vi "Save_Single_Timetrace.vi"(1 "Headers":T1, 2 "Put each block into separate file":bool, 3 "Precision":i16=2, 7 "Index":i32, 9 "File Extension":string=".xls", 12 "Leave space between blocks?":bool, 14 "Separation Character":enum16{"Tab", "Comma"}(ring)) -> (4 "Plug in titles":string[](array[string]), 8 "Plug in values":string[](array[string]))   [LabVIEW 2021]
uses:
  Controls/Inst_type.ctl
  File/File Update Cluster.ctl
  Globals/Meas_global.vi
  Controls/File Header mode.ctl
panel:
  out "Output:Data File:Location":string
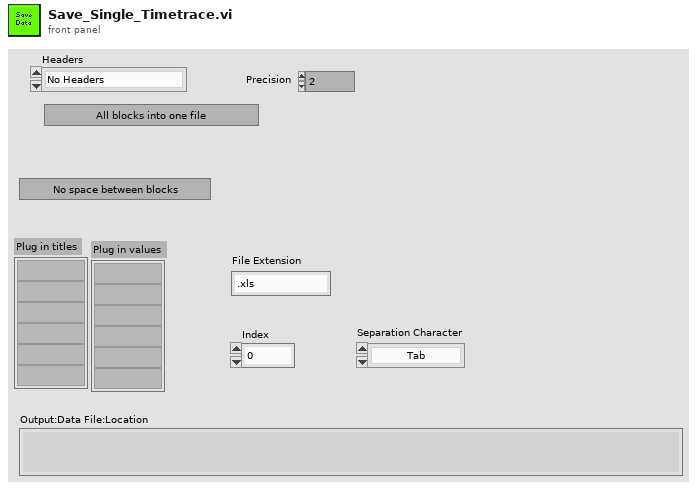
[diagram p1: front panel]
types:
  T1 = typedef "File Header mode.ctl" = enum16{"No Headers", "Headers in All files", "Separate Header File"}
  T2 = typedef "Analysis_info_cluster.ctl" = cluster{"Colour":u32, "Inst type":T3, "Inst name":string, "Symbol":string, "Code name":string, "Extra Info":string, "Inst Array":T4, "Extra Titles":string[], "Extra Values":string[], "U":dbl, "u^2":dbl, "u^3":dbl, "u^4":dbl, "Skew_u":dbl, "Kurt_u":dbl, "Sd Error in Mean":dbl, "% u'/U":dbl, "X":dbl, "Y":dbl, "Z":dbl, "Timescale integral Estimate":dbl, "Sd Error in Variance":dbl, "Calib File":path, "Calib Constants":dbl[], "Output Position":bool, "Stats":enum16{"None", "Basic", "Full"}, "Av Sampling Rate":dbl, "Av No of Samples":dbl, "Total Meas Time (s)":dbl, "ADAM Ch Name":string, "Max value":dbl, "Min value":dbl, "Req Sample Rate Hz":dbl, "Sync Delay Time (s)":dbl, "Ch No":i16, "Device":string, "Use Latest Calib":bool, "Port":string, "Metadata Ch Names":string[], "Metadata Ch Values":string[], "Label":string}
  T3 = typedef "Inst_type.ctl" = enum16{"Raw voltage", "Raw with zero offsetting", "Propeller anemometer", "Pressure Transducer", "Pitot-static tube", "Hot wire", "Cross wire 1", "Cross wire 2", "Generic Linear", "Generic Polynomial", "Generic BackPoly", "Fast FID", "Thermocouple", "Cold wire", "Pulsed Wire", "LDA Vel", "LDA Tran time", "LDA Arr time", "Microphone"}
  T4 = typedef "Instrument_Array.ctl" = enum16{"PWA", "LDA", "Analogue"}
  T5 = typedef "File Update Cluster.ctl" = cluster{"File Path":path, "Rows to Add":i32[], "Extra Ch Names":string[], "Extra Ch Values":string[], "Initial Header String":string, "Separation Character":enum16{"Tab", "Comma"}}
  T6 = typedef "Time_Trace_Cluster.ctl" = cluster{"Weighting":dbl[], "Voltage":dbl[], "Eng Values":dbl[]}
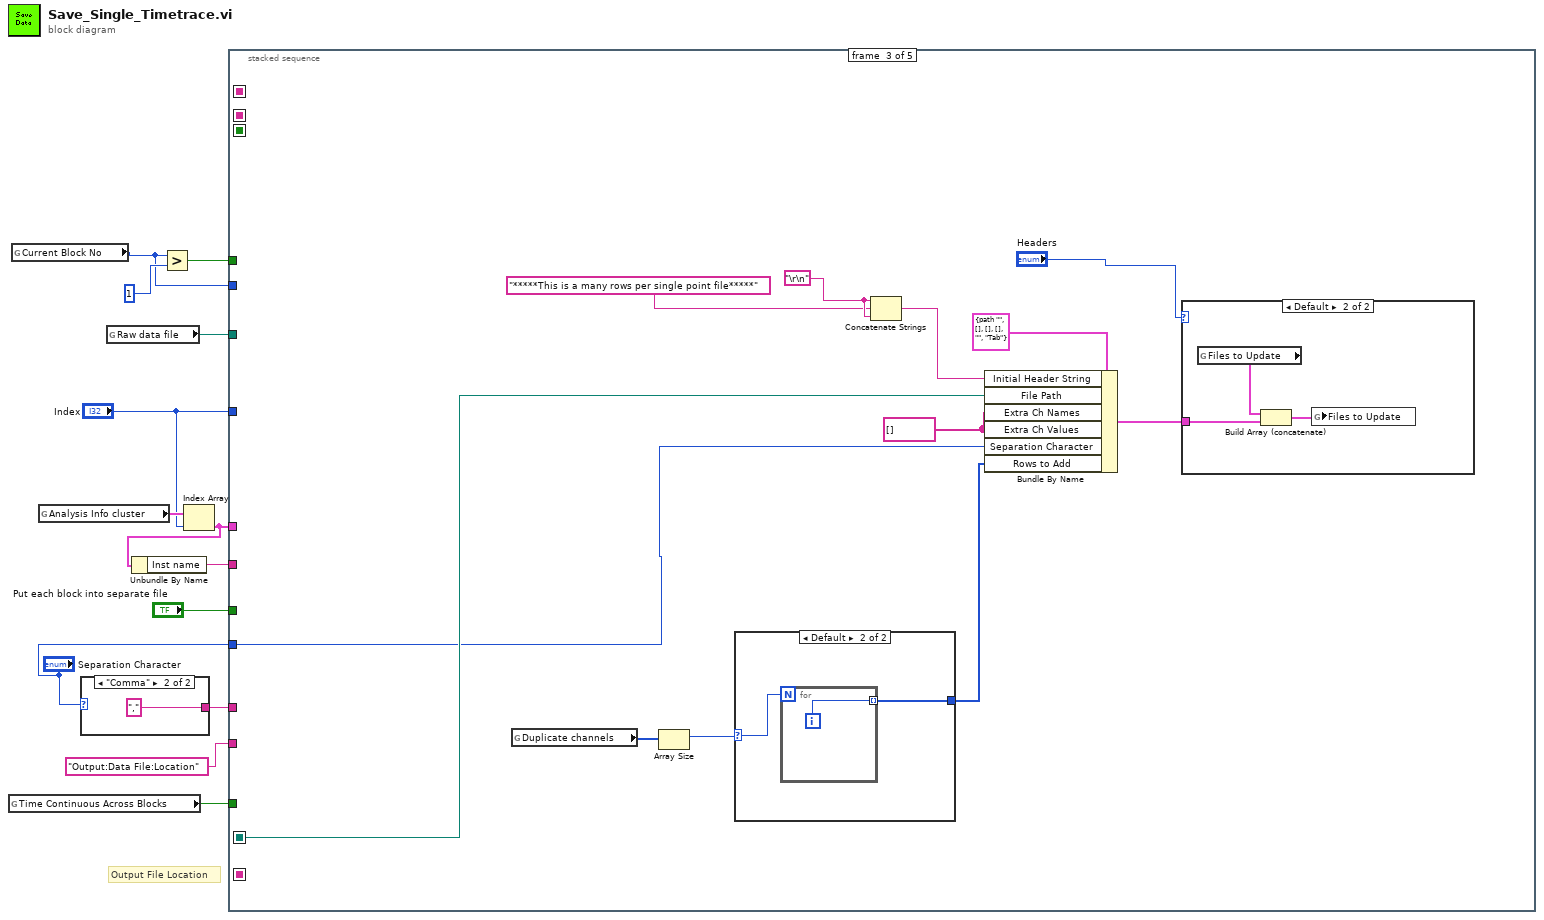
[diagram p0: block diagram]
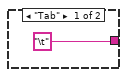
[diagram p2: hidden frame]
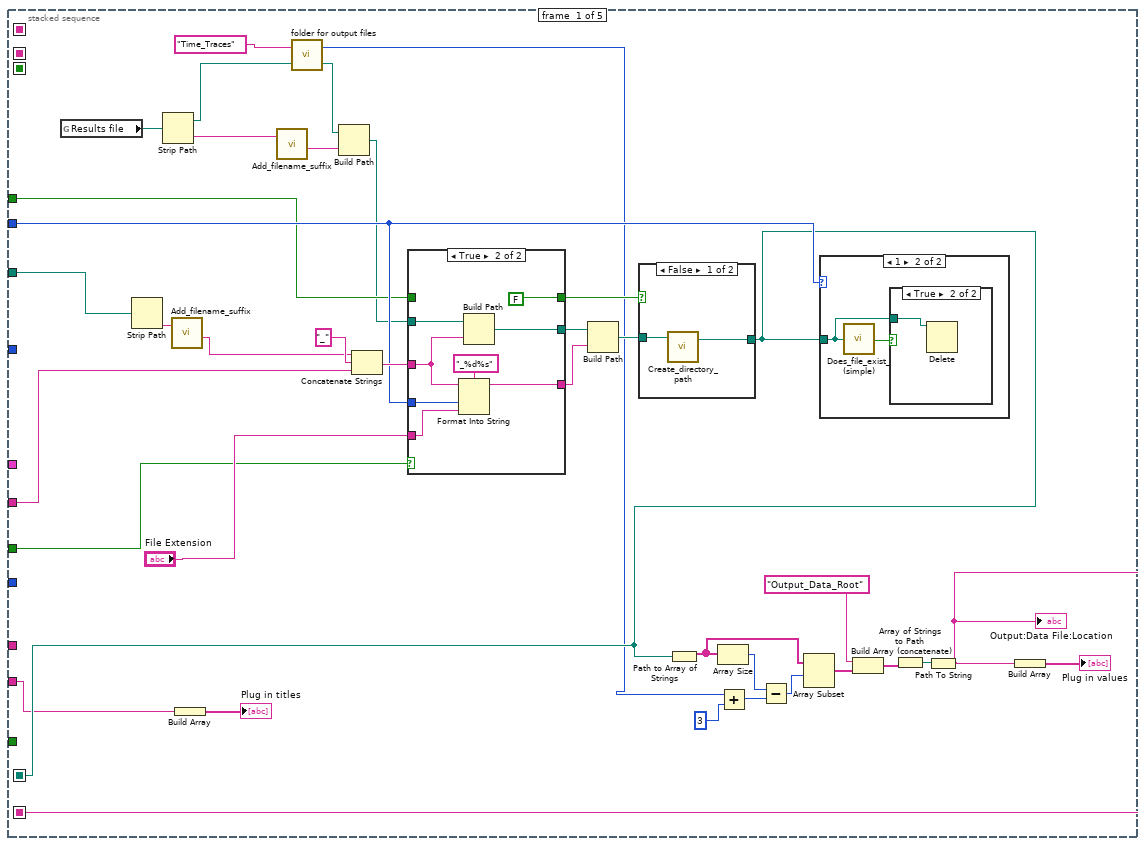
[diagram p3: hidden frame]
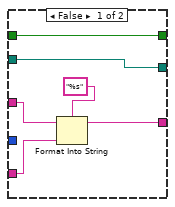
[diagram p6: hidden frame]
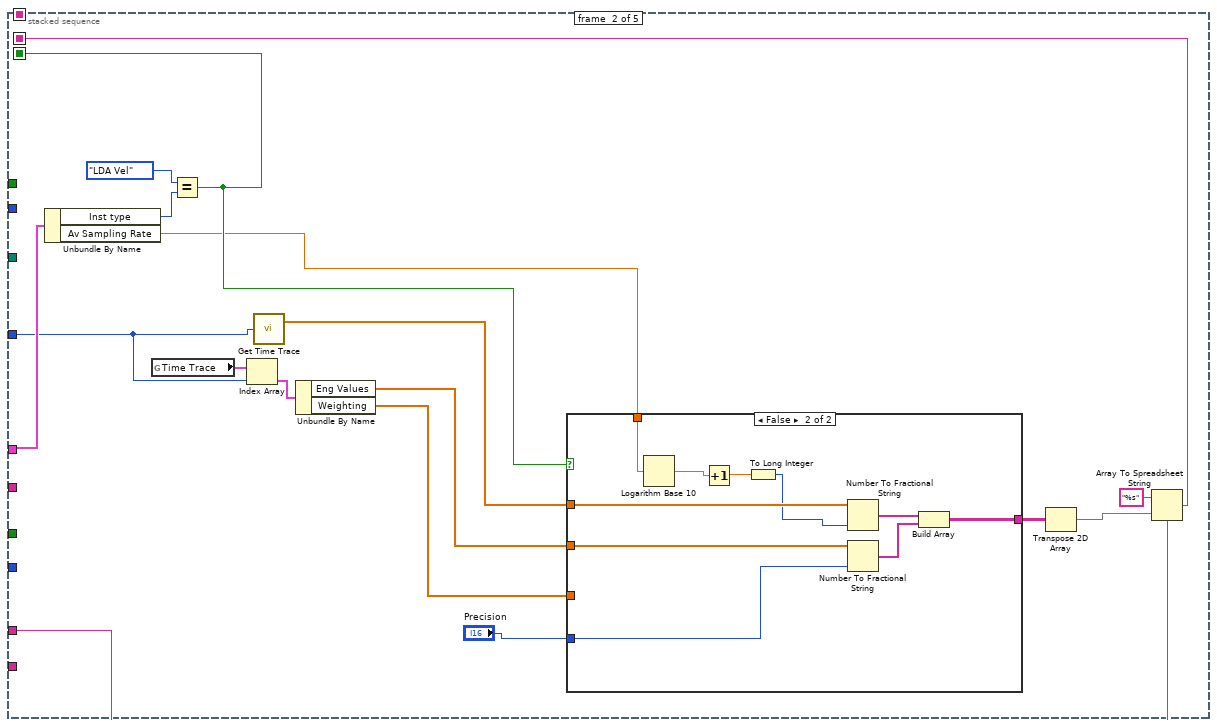
[diagram p8: hidden frame]
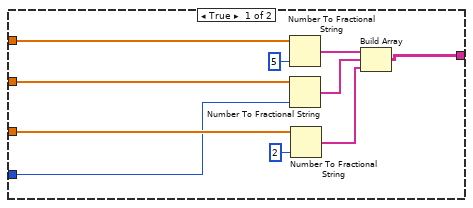
[diagram p9: hidden frame]
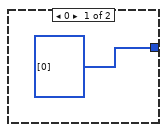
[diagram p11: hidden frame]
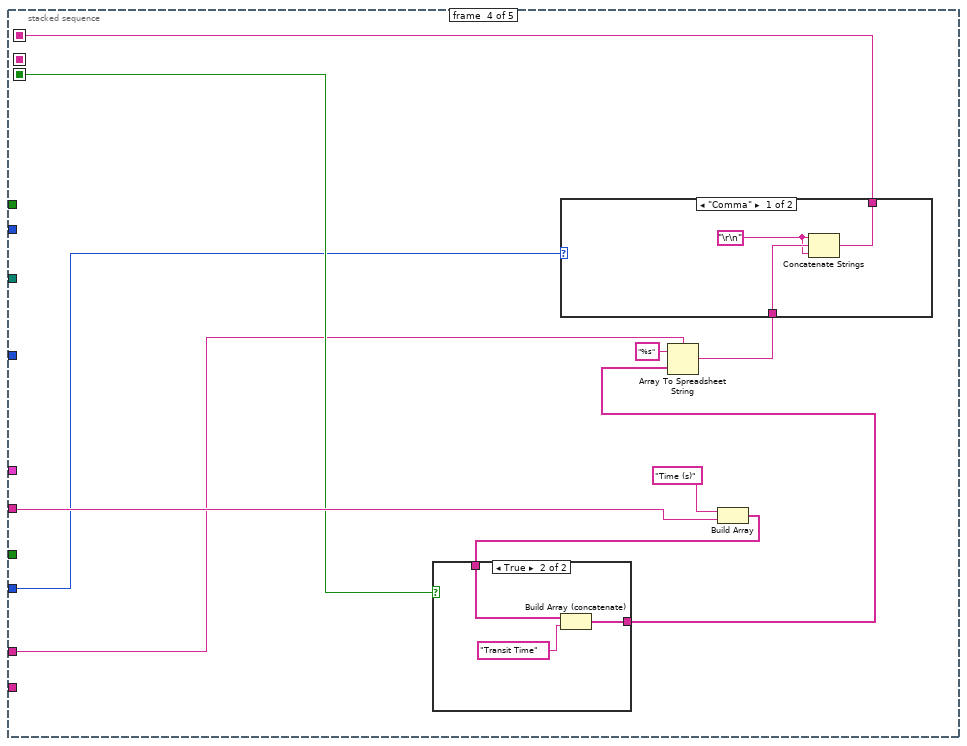
[diagram p12: hidden frame]
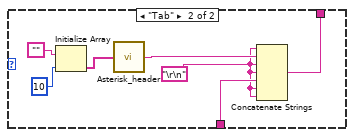
[diagram p14: hidden frame]
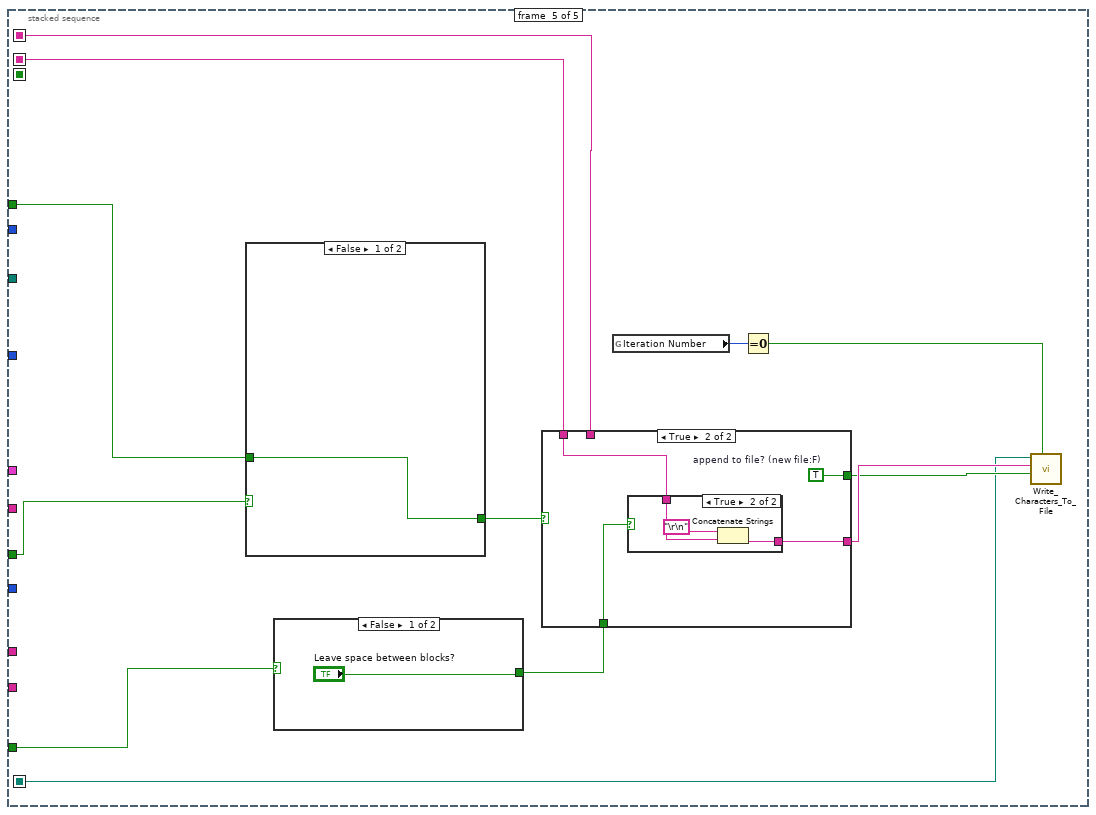
[diagram p15: hidden frame]
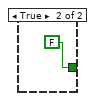
[diagram p16: hidden frame]
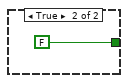
[diagram p17: hidden frame]
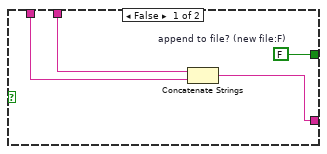
[diagram p18: hidden frame]
diagram:
  # "Output File Location"
  n1 = global read "Meas_global.vi" "Time Continuous Across Blocks"() -> (w2:bool)
  n2 = global read "Meas_global.vi" "Current Block No"() -> (w7:i32)
  n3 = global read "Meas_global.vi" "Analysis Info cluster"() -> (w13:T2[])
  n4 = case shown="\"Comma\"" "Separation Character" {
    tunnel: ["\t" ("Separation Character 2") ","] -> w11
    frame "Tab" {
    }
    frame "Comma" {
    }
  }
  n5 = global read "Meas_global.vi" "Raw data file"() -> (w9:path)
  n6 = Greater?(x=w7, y=1) -> (0:w6:bool)
  n7 = Index Array(array=w13, index="Index") -> (element=w5:T2)
  n8 = Unbundle By Name(w5) -> ("Inst name"=w4:string)
  n9 = stacked-sequence {
    seq-local: [_ w78 _ _ _] -> [_ _ _ _ w153]
    seq-local: [_ w77 _ _ _] -> [_ _ _ w133 _]
    seq-local: [w22 _ _ _ _] -> [_ _ _ _ _]
    seq-local: [w21 _ _ _ _] -> [_ _ w111 _ w152]
    seq-local: [_ _ _ w130 _] -> [_ _ _ _ w154]
    tunnel: w5 -> [_ w88 _ _ _]
    tunnel: "Index" -> [_ w73 _ _ _]
    tunnel: w11 -> [_ w79 _ w128 _]
    tunnel: "Output:Data File:Location" -> [w16 _ _ _ _]
    tunnel: w9 -> [w43 _ _ _ _]
    tunnel: w7 -> [w25 _ _ _ _]
    tunnel: w6 -> [w24 _ _ _ w157]
    tunnel: w4 -> [w20 _ _ w134 _]
    tunnel: "Put each block into separate file" -> [w19 _ _ _ w156]
    tunnel: w2 -> [_ _ _ _ w155]
    tunnel: "Separation Character" -> [_ _ w110 w129 _]
    frame #0 {
      n10 = global read "Meas_global.vi" "Results file"() -> (w39:path)
      n11 = Strip Path(path=w43) -> (name=w44:string)  [unwired: 1 out]
      n12 = Strip Path(path=w39) -> (stripped path=w38:path, name=w40:string)
      n13 = call "Add_filename_suffix.vi"("Filename"=w44) -> ("Base name"=w42:string)  [unwired: 1 in, 3 out]
      n14 = Build Array(w16) -> (→"Plug in titles":string[])
      n15 = call "Add_filename_suffix.vi"("Filename"=w40) -> ("Base name"=w41:string)  [unwired: 1 in, 3 out]
      n16 = call "folder for output files.vi"("results folder"=w38, "folder name"="Time_Traces" ("name or relative path")) -> ("appended path"=w36:path, "Plug_in folder depth"=w18:i32)
      n17 = Build Path(base path=w36, name or relative path=w41) -> (appended path=w23:path)
      n18 = Concatenate Strings(w42, "_" ("format string"), w20) -> (w46:string)
      n19 = case shown="True" w19 {
        tunnel: w46 -> [w57 w64]
        tunnel: w25 -> [_ w62]
        tunnel: [w56 w67] -> w51
        tunnel: w24 -> [w60 _]
        tunnel: [w60 FALSE] -> w50
        tunnel: [w59 w63] -> w49
        tunnel: w23 -> [w59 w65]
        tunnel: "File Extension" -> [w55 w61]
        frame False {
          n20 = Format Into String(format string="%s", initial string=w57, w55) -> (resulting string=w56:string)  [unwired: 1 in, 1 out]
        }
        frame True {
          n21 = Format Into String(format string="_%d%s", initial string=w64, w62, w61) -> (resulting string=w67:string)  [unwired: 1 in, 1 out]
          n22 = Build Path(base path=w65, name or relative path=w64) -> (appended path=w63:path)
        }
      }
      n23 = Build Path(base path=w49, name or relative path=w51) -> (appended path=w48:path)
      n24 = case shown="False" w50 {
        tunnel: w48 -> [w70 w71]
        tunnel: [w69 w71] -> w21
        frame False {
          n25 = call "Create_directory_path.vi"("Path name"=w70) -> ("Path name Out"=w69:path)  [unwired: 2 in, 1 out]
        }
        frame True {
        }
      }
      n26 = Path to Array of Strings(0:w21) -> (2:w27:string[])  [unwired: 1 out]
      n27 = Array Size(array=w27) -> (size(s)=w26:i32)
      n28 = Add(x=w18, y=3) -> (x+y=w35:i32)
      n29 = Subtract(x=w26, y=w35) -> (x-y=w28:i32)
      n30 = Array Subset(array=w27, index=w28) -> (w30:string[])  [unwired: 1 in]
      n31 = case shown="1" w25 {
        tunnel: w21 -> [_ w52]
        frame Default {
        }
        frame 1 {
          n32 = call "Does_file_exist_(simple).vi"("Pathname"=w52) -> ("exists?"=w53:bool)
          n33 = case shown="True" w53 {
            tunnel: w52 -> [_ w54]
            frame False {
            }
            frame True {
              n34 = Delete(path (use dialog)=w54) -> ()  [unwired: 4 in, 3 out]
            }
          }
        }
      }
      n35 = Build Array (concatenate)("Output_Data_Root", w30) -> (w31:string[])
      n36 = Array of Strings to Path(0:w31) -> (2:w29:path)  [unwired: 1 in]
      n37 = Path To String(path=w29) -> (string=w22:string)
      "Output:Data File:Location" <- w22
      n38 = Build Array(w22) -> (→"Plug in values":string[])
    }
    frame #1 {
      n39 = Unbundle By Name(w88) -> ("Inst type"=w85:T3, "Av Sampling Rate"=w74:dbl)
      n40 = global read "Meas_global.vi" "Time Trace"() -> (w87:T6[])
      n41 = Equal?(x=Inst_type."LDA Vel" ("Inst type"), y=w85) -> (x = y?=w77:bool)
      n42 = Index Array(array=w87, index=w73) -> (element=w86:T6)
      n43 = call "Get Time Trace.vi"("Channel Index"=w73) -> ("Time (s)"=w72:dbl[])  [unwired: 1 out]
      n44 = Unbundle By Name(w86) -> ("Eng Values"=w83:dbl[], "Weighting"=w82:dbl[])
      n45 = case shown="False" w77 {
        tunnel: [w98 w108] -> w80
        tunnel: w72 -> [w96 w106]
        tunnel: w83 -> [w95 w105]
        tunnel: w82 -> [w93 _]
        tunnel: "Precision" -> [w90 w103]
        tunnel: w74 -> [_ w100]
        frame True {
          n46 = Number To Fractional String(number=w96, precision (6)=i16 5) -> (F-format string=w94:string[])  [unwired: 2 in]
          n47 = Number To Fractional String(number=w95, precision (6)=w90) -> (F-format string=w97:string[])  [unwired: 2 in]
          n48 = Number To Fractional String(number=w93, precision (6)=i16 2) -> (F-format string=w92:string[])  [unwired: 2 in]
          n49 = Build Array(w94, w97, w92) -> (w98:string[][])
        }
        frame False {
          n50 = Logarithm Base 10(1:w100) -> (0:w101:dbl)
          n51 = Increment(x=w101) -> (x+1=w102:dbl)
          n52 = To Long Integer(number=w102) -> (32bit integer=w99:i32)
          n53 = Number To Fractional String(number=w106, precision (6)=w99) -> (F-format string=w104:string[])  [unwired: 2 in]
          n54 = Number To Fractional String(number=w105, precision (6)=w103) -> (F-format string=w107:string[])  [unwired: 2 in]
          n55 = Build Array(w104, w107) -> (w108:string[][])
        }
      }
      n56 = Transpose 2D Array(2D array=w80) -> (transposed array=w75:string[][])
      n57 = Array To Spreadsheet String(delimiter (Tab)=w79, array=w75, 3:"%s" ("format string")) -> (spreadsheet string=w78:string)
    }
    frame #2 {
      w113 = string[] [] ("Extra Ch Names")
      w120 = "\r\n"
      n58 = global read "Meas_global.vi" "Duplicate channels"() -> (w116:i32[])
      n59 = Array Size(array=w116) -> (size(s)=w117:i32)
      n60 = case shown="Default" w117 {
        selector: w117 -> [_ w126]
        tunnel: [i32[] [0] ("Rows to Add") w125] -> w118
        frame 0 {
        }
        frame Default {
          n61 = for {
            N: w126 -> [_]
            tunnel: [w127] -> w125 mode=indexing
            i -> [w127]
          }
        }
      }
      n62 = Concatenate Strings(w120, "*****This is a many rows per single point file*****", w120) -> (w112:string)
      n63 = Bundle By Name(cluster=T5 {"File Path"=path "", "Rows to Add"=[], "Extra Ch Names"=[], "Extra Ch Values"=[], "Initial Header String"="", "Separation Character"=enum."Tab"} ("File to Update"), "Initial Header String"=w112, "File Path"=w111, "Extra Ch Names"=w113, "Extra Ch Values"=w113, "Separation Character"=w110, "Rows to Add"=w118) -> (w115:T5)
      n64 = case shown="Default" "Headers" {
        tunnel: w115 -> [_ w122]
        frame "No Headers" {
        }
        frame Default {
          n65 = global read "Meas_global.vi" "Files to Update"() -> (w121:T5[])
          n66 = Build Array (concatenate)(w121, w122) -> (w123:T5[])
          n67 = global write "Meas_global.vi" "Files to Update"(w123) -> ()
        }
      }
    }
    frame #3 {
      n68 = Build Array("Time (s)", w134) -> (w132:string[])
      n69 = case shown="True" w133 {
        tunnel: w132 -> [w138 w140]
        tunnel: [w138 w139] -> w131
        frame False {
        }
        frame True {
          n70 = Build Array (concatenate)(w140, "Transit Time") -> (w139:string[])
        }
      }
      n71 = Array To Spreadsheet String(delimiter (Tab)=w128, array=w131, 3:"%s" ("format string")) -> (spreadsheet string=w136:string)
      n72 = case shown="\"Comma\"" w129 {
        tunnel: [w144 w151] -> w130
        tunnel: w136 -> [w143 w150]
        frame "Comma" {
          w142 = "\r\n"
          n73 = Concatenate Strings(w142, w143, w142) -> (w144:string)
        }
        frame "Tab" {
          w145 = "\r\n"
          n74 = Initialize Array("", 10) -> (w147:string[])
          n75 = call "Asterisk_header.vi"("Channel names"=w147) -> ("Header string"=w146:string)
          n76 = Concatenate Strings(w145, w146, w145, w145, w150, w145, w145) -> (w151:string)
        }
      }
    }
    frame #4 {
      n77 = case shown="False" w156 {
        tunnel: [w164 FALSE] -> w163
        tunnel: w157 -> [w164 _]
        frame False {
        }
        frame True {
        }
      }
      n78 = case shown="False" w155 {
        tunnel: ["Leave space between blocks?" FALSE] -> w162
        frame False {
        }
        frame True {
        }
      }
      n79 = case shown="True" w163 {
        tunnel: [w168 w175] -> w159
        tunnel: [w171 w174] -> w158
        tunnel: w162 -> [_ w173]
        tunnel: w154 -> [w170 _]
        tunnel: w153 -> [w169 w172]
        frame False {
          w171 = FALSE  # append to file? (new file:F)
          n80 = Concatenate Strings(w170, w169) -> (w168:string)
        }
        frame True {
          w174 = TRUE  # append to file? (new file:F)
          n81 = case shown="True" w173 {
            tunnel: [w176 w179] -> w175
            tunnel: w172 -> [w176 w178]
            frame False {
            }
            frame True {
              n82 = Concatenate Strings("\r\n", w178) -> (w179:string)
            }
          }
        }
      }
      n83 = global read "Meas_global.vi" "Iteration Number"() -> (w160:i32)
      n84 = Equal To 0?(x=w160) -> (x = 0?=w161:bool)
      n85 = call "Write_Characters_To_File.vi"("file path (dialog if empty)"=w152, "advisory dialog? (display:T)"=w161, "character string"=w159, "append to file? (new file:F)"=w158) -> ()  [unwired: 1 in, 4 out]
    }
  }
